vi "GetAppOutput.vi"(8 "error in (no error)":errorcluster, 11 "RingdownPlugin in":refnum<class "EraPlugin.lvclass">) -> (0 "error out":errorcluster, 3 "RingdownPlugin out":refnum<class "EraPlugin.lvclass">)   [LabVIEW 2017, in "AppPlugins.lvlib" / "ERAPlugin.lvclass"]
uses:
  EraPlugin.lvclass
  C:/dev/Work/PARTF/Modules/AppPlugins/AppPluginBaseClass/AppPluginsBase.lvclass
  TypeDef/ERAOutput.ctl
  EraPlugin.lvclass/EraPlugin.ctl
  <vilib>/Analysis/7linalg.llb/Eigenvalue and Vectors Output Option.ctl
  Accessors/Read RingdownConfig.vi
  <vilib>/Analysis/7linalg.llb/Real Eigenvalues and Vectors.vi
  <vilib>/Analysis/Matrix/Numeric/Conversions/Array To Matrix - CA2.vi
  <vilib>/Analysis/7linalg.llb/Solve Complex Linear Equations (single right hand).vi
  <vilib>/Analysis/NI_AALPro.lvlib
  LabVIEW/mode-estimation/src/Mode Estimation/Mode Estimation.lvlib
  <vilib>/Analysis/Matrix/NI_Matrix.lvlib
panel:
  out "Damping ratio":dbl[](array[numeric])
  out "Output Parameters":T1
  out "Time of process":dbl
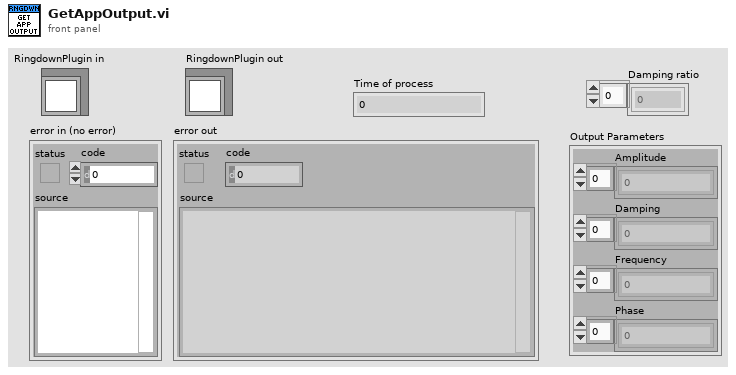
[diagram p1: front panel]
types:
  T1 = cluster{"Amplitude":dbl[], "Damping":dbl[], "Frequency":dbl[], "Phase":dbl[]}
  T2 = typedef "AppPlugins.lvlib/ERAPlugin.lvclass/ERAOutput.ctl" = cluster{"FramesPerSecond":dbl, "RingdownParameters":cluster{"Amplitude":dbl[], "Damping":dbl[], "Frequency":dbl[], "Phase":dbl[]}, "ReportingTime":dbl, "DataSize":u32, "InputSignal":dbl[]}
  T3 = typedef "AppPlugins.lvlib/ERAPlugin.lvclass/RingdownConfig.ctl" = cluster{"Config":cluster{"p_SysOdr":i32, "dThres":dbl, "Preproc":cluster{"order":i32, "f_lo":dbl, "f_hi":dbl, "R_down":i32}}, "V index":i32, "I index":i32, "PosSeq":bool}
  T4 = cluster{"order":i32, "f_lo":dbl, "f_hi":dbl, "R_down":i32}
  T5 = typedef "NI_Matrix.lvlib/RealMatrix.ctl" = dbl[][]
  T6 = typedef "NI_AALPro.lvlib/Eigenvalue and Vectors Output Option.ctl" = i32
  T7 = cluster{"Damping":dbl, "Frequency":dbl, "Re(Pole)":dbl, "Im(Pole)":dbl}[]
  T8 = typedef "NI_Matrix.lvlib/ComplexMatrix.ctl" = cdb[][]
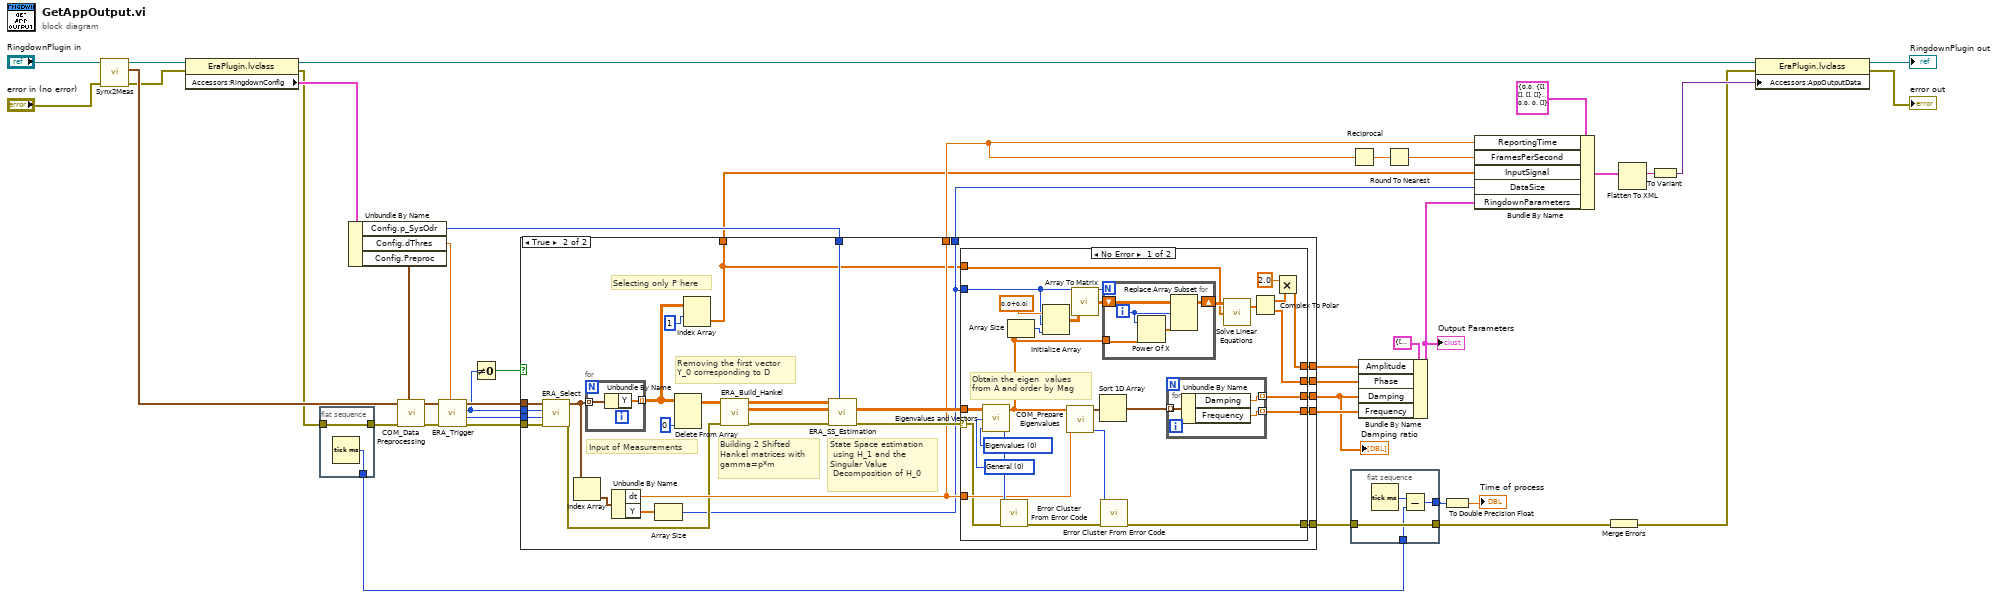
[diagram p0: block diagram]
diagram:
  n1 = call "Synx2Meas.vi"("error in (no error)"="error in (no error)", "RingdownPlugin in"="RingdownPlugin in") -> ("error out"=w4:errorcluster, "Measurements"=w27:waveform(dbl)[], "RingdownPlugin out"=w5:refnum<class "EraPlugin.lvclass">)  [unwired: 7 in]
  n2 = property class="EraPlugin.lvclass"(reference=w5, error in=w4) -> (reference out=w2:refnum<class "EraPlugin.lvclass">, error out=w3:errorcluster, "Accessors:RingdownConfig"=w29:T3)
  n3 = flat-sequence {
    tunnel: [w44] -> w15
    tunnel: [w43] -> w14
    tunnel: w3 -> [w43]
    frame #0 {
      n4 = Tick Count (ms)() -> (millisecond timer value=w44:u32)
    }
  }
  n5 = Unbundle By Name(w29) -> ("Config.p_SysOdr"=w30:i32, "Config.dThres"=w26:dbl, "Config.Preproc"=w1:T4)
  n6 = call "COM_Data Preprocessing.vi"("Parameters"=w1, "error in"=w14, "Waveforms IN"=w27) -> ("error out"=w25:errorcluster, "Waveforms OUT"=w28:waveform(dbl)[])  [unwired: 7 in]
  n7 = call "ERA_Trigger.vi"("Threshold"=w26, "Error In"=w25, "Data In"=w28) -> ("Error Out"=w21:errorcluster, "Ind_end"=w20:i32, "Ind_begin"=w19:i32, "Data Out"=w22:waveform(dbl)[])  [unwired: 4 in, 1 out]
  n8 = Not Equal To 0?(x=w19) -> (x != 0?=w18:bool)
  n9 = case shown="True" w18 {
    tunnel: w30 -> [_ w66]
    tunnel: [_ w63] -> w24
    tunnel: [_ w49] -> w23
    tunnel: [w45 w62] -> w17
    tunnel: w22 -> [_ w61]
    tunnel: w21 -> [w45 w58]
    tunnel: w20 -> [_ w57]
    tunnel: w19 -> [_ w56]
    tunnel: [_ w55] -> w7
    tunnel: [_ w54] -> w11
    tunnel: [_ w51] -> w10
    tunnel: [_ w48] -> w9
    tunnel: [_ w47] -> w8
    frame False {
    }
    frame True {
      # "Selecting only P here"
      # "State Space estimation\n using H_1 and the \nSingular Value\n Decomposition of H_0"
      # "Building 2 Shifted \nHankel matrices with\ngamma=p*m"
      # "Removing the first vector\nY_0 corresponding to D"
      # "Input of Measurements"
      n10 = call "ERA_Select.vi"("Error In"=w58, "Ind_end"=w57, "Ind_begin"=w56, "Data In"=w61) -> ("Error Out"=w59:errorcluster, "Data Out"=w60:waveform(dbl)[])  [unwired: 6 in]
      n11 = Index Array(array=w60) -> (element=w53:waveform(dbl))  [unwired: 1 in]
      n12 = for {
        tunnel: w60 -> [w108] mode=indexing
        tunnel: [w107] -> w50 mode=indexing
        n13 = Unbundle By Name(w108) -> ("Y"=w107:dbl[])
      }
      n14 = Unbundle By Name(w53) -> ("dt"=w63:dbl, "Y"=w52:dbl[])
      n15 = Array Size(array=w52) -> (size(s)=w51:i32)
      n16 = Delete From Array(array=w50, index (col)=0 ("disabled index (col)")) -> (array with subset deleted=w70:dbl[][])  [unwired: 2 in, 1 out]
      n17 = Index Array(array=w50, index (row)=1 ("disabled index (col)")) -> (element=w49:dbl[])  [unwired: 1 in]
      n18 = call "ERA_Build_Hankel.vi"("error in (no error)"=w59, "Measurements"=w70) -> ("error out"=w65:errorcluster, "H_1"=w68:T5, "H_0"=w69:T5)  [unwired: 7 in]
      n19 = call "ERA_SS_Estimation.vi"("Order Index"=w66, "Error In"=w65, "H_1"=w68, "H_0"=w69) -> ("Error Out"=w64:errorcluster, "A"=w67:T5)  [unwired: 4 in, 2 out]
      n20 = case shown="No Error" w64 {
        selector: w64 -> [w85 w106]
        tunnel: w67 -> [w95 _]
        tunnel: w63 -> [w91 _]
        tunnel: [w92 w106] -> w62
        tunnel: [w87 _] -> w55
        tunnel: [w86 _] -> w54
        tunnel: w51 -> [w72 _]
        tunnel: w49 -> [w79 _]
        tunnel: [w77 _] -> w48
        tunnel: [w74 _] -> w47
        frame No Error {
          w96 = T6 0 items=["Eigenvalues", "Eigenvalues & Vectors"] ("output option")
          w97 = 0 items=["General", "Symmetric"] ("matrix type")
          # "Obtain the eigen  values \nfrom A and order by Mag"
          n21 = call-poly <vilib>:"Eigenvalues and Vectors.vi"("output option"=w96, "matrix type"=w97, "Input Matrix"=w95) -> ("error"=w94:i32, "Eigenvalues"=w83:cdb[])  [unwired: 1 out]
          n22 = call <vilib>:"Error Cluster From Error Code.vi"("error in (no error)"=w85, "error code (0)"=w94) -> ("error out"=w93:errorcluster)  [unwired: 7 in]
          n23 = Array Size(array=w83) -> (size(s)=w73:i32)
          n24 = Initialize Array(cdb 0.0+0.0i ("element"), w72, w73) -> (w82:cdb[][])
          n25 = call "COM_Prepare Eigenvalues.vi"("dt"=w91, "Eigenvalues"=w83) -> ("error"=w90:i32, "Modes OUT"=w89:T7)  [unwired: 8 in]
          n26 = call-poly <vilib>:"Array To Matrix.vi"("Complex 2D Array"=w82) -> ("Complex Matrix"=w81:T8)
          n27 = Sort 1D Array(array=w89) -> (sorted array=w88:T7)
          n28 = call <vilib>:"Error Cluster From Error Code.vi"("error in (no error)"=w93, "error code (0)"=w90) -> ("error out"=w92:errorcluster)  [unwired: 7 in]
          n29 = for {
            N: w72 -> [_]
            shift-right: [w101] -> w80
            shift-left: w81 -> [w102]
            tunnel: w83 -> [w100]
            i -> [w99]
            n30 = Power Of X(1:w100, 2:w99) -> (0:w98:cdb[])
            n31 = Replace Array Subset(array=w102, new element=w98, index (row)=w99) -> (w101:T8)  [unwired: 1 in]
          }
          n32 = for {
            tunnel: w88 -> [w105] mode=indexing
            tunnel: [w104] -> w87 mode=indexing
            tunnel: [w103] -> w86 mode=indexing
            n33 = Unbundle By Name(w105) -> ("Damping"=w104:dbl, "Frequency"=w103:dbl)
          }
          n34 = call-poly <vilib>:"Solve Linear Equations.vi"("Known Vector"=w79, "Input Matrix"=w80) -> ("Solution Vector"=w76:cdb[])  [unwired: 1 in, 1 out]
          n35 = Complex To Polar(r * e^(i*theta)=w76) -> (r=w75:dbl[], theta=w74:dbl[])
          n36 = Multiply(x=2.0, y=w75) -> (x*y=w77:dbl[])
        }
        frame Error {
        }
      }
    }
  }
  "Damping ratio" <- w7
  n37 = Reciprocal(x=w24) -> (1/x=w40:dbl)
  n38 = flat-sequence {
    tunnel: w17 -> [w112]
    tunnel: [w112] -> w16
    tunnel: w15 -> [w110]
    tunnel: [w109] -> w13
    frame #0 {
      n39 = Tick Count (ms)() -> (millisecond timer value=w111:u32)
      n40 = Subtract(x=w111, y=w110) -> (x-y=w109:u32)
    }
  }
  n41 = Bundle By Name(cluster=T1 {"Amplitude"=[], "Damping"=[], "Frequency"=[], "Phase"=[0.0, 0.0, 0.0, 0.0, 0.0, 0.0, 0.0, 0.0, 0.0, 0.0, 0.0, 0.0, 0.0, 0.0, 0.0, 0.0]} ("RingdownParameters"), "Amplitude"=w9, "Phase"=w8, "Damping"=w7, "Frequency"=w11) -> (w6:T1)
  "Output Parameters" <- w6
  n42 = Round To Nearest(number=w40) -> (nearest integer value=w39:dbl)
  n43 = To Double Precision Float(number=w13) -> (double precision float=→"Time of process":dbl)
  n44 = Bundle By Name(cluster=T2 {"FramesPerSecond"=0.0, "RingdownParameters"={"Amplitude"=[], "Damping"=[], "Frequency"=[], "Phase"=[]}, "ReportingTime"=0.0, "DataSize"=0, "InputSignal"=[]} ("RingdownOutput"), "ReportingTime"=w24, "FramesPerSecond"=w39, "InputSignal"=w23, "DataSize"=w10, "RingdownParameters"=w6) -> (w34:T2)
  n45 = Merge Errors(w16) -> (w31:errorcluster)
  n46 = Flatten To XML(anything=w34) -> (xml string=w33:string)
  n47 = To Variant(anything=w33) -> (Variant=w32:variant)
  n48 = property class="EraPlugin.lvclass"(reference=w2, error in=w31, "Accessors:AppOutputData"=w32) -> (reference out=→"RingdownPlugin out":refnum<class "EraPlugin.lvclass">, error out=→"error out":errorcluster)
